vi "Interpret Opcode.vi"(10 "Opcode":u8 format="%x", 11 "Disassembler in":refnum<class "Disassembler.lvclass">) -> (1 "Addressing Mode":T2=enum."Immediate", 2 "Mnemonic":T1=enum."NOP", 3 "Disassembler out":refnum<class "Disassembler.lvclass">)   [LabVIEW 2021, in "Disassembler.lvclass"]
uses:
  Disassembler.lvclass
  Addressing Mode.ctl
  Menmonic.ctl
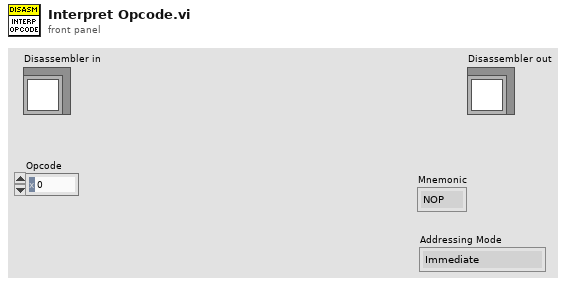
[diagram p1: front panel]
types:
  T1 = typedef "Disassembler.lvclass/Menmonic.ctl" = enum16{"Undefined", "ADC", "AND", "ASL", "BCC", "BCS", "BEQ", "BIT", "BMI", "BNE", "BPL", "BRK", "BVC", "BVS", "CLC", "CLD", "CLI", "CLV", "CMP", "CPX", "CPY", "DEC", "DEX", "DEY", "EOR", "INC", "INX", "INY", "JMP", "JSR", "LDA", "LDX", "LDY", "LSR", "NOP", "ORA", "PHA", "PHP", "PLA", "PLP", "ROL", "ROR", "RTI", "RTS", "SBC", "SEC", "SED", "SEI", "STA", "STX", "STY", "TAX", "TAY", "TSX", "TXA", "TXS", "TYA"}
  T2 = typedef "Disassembler.lvclass/Addressing Mode.ctl" = enum16{"Undefined", "Zero Page,Y", "Zero Page,X", "Zero Page", "Relative", "(indirect,X)", "(indirect),Y", "Implicit", "Immediate", "Accumulator", "Absolute,Y", "Absolute,X", "Absolute", "Indirect"}
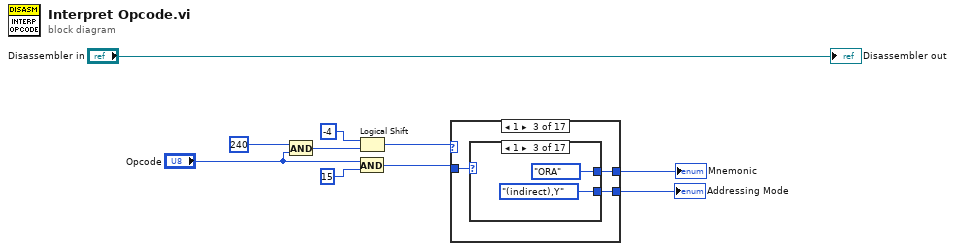
[diagram p0: block diagram]
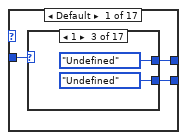
[diagram p2: hidden frame]
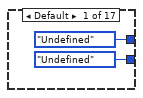
[diagram p3: hidden frame]
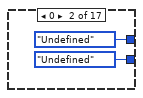
[diagram p4: hidden frame]
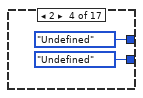
[diagram p5: hidden frame]
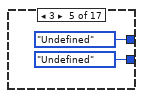
[diagram p6: hidden frame]
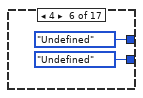
[diagram p7: hidden frame]
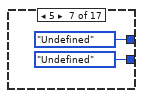
[diagram p8: hidden frame]
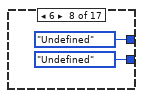
[diagram p9: hidden frame]
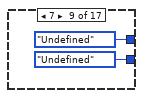
[diagram p10: hidden frame]
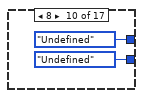
[diagram p11: hidden frame]
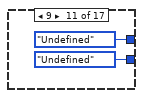
[diagram p12: hidden frame]
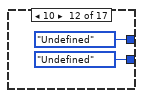
[diagram p13: hidden frame]
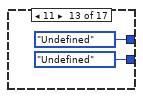
[diagram p14: hidden frame]
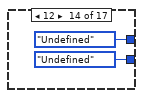
[diagram p15: hidden frame]
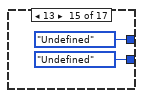
[diagram p16: hidden frame]
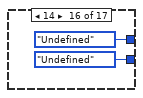
[diagram p17: hidden frame]
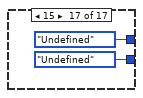
[diagram p18: hidden frame]
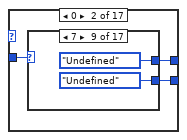
[diagram p19: hidden frame]
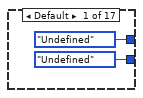
[diagram p20: hidden frame]
diagram:
  n1 = And(x=u8 240, y="Opcode") -> (x .and. y?=w8:u8)
  n2 = Logical Shift(y=i8 -4, x=w8) -> (x << y=w4:u8)
  n3 = And(x="Opcode", y=u8 15) -> (x .and. y?=w3:u8)
  n4 = case shown="1" w4 {
    tunnel: w3 -> [w13 w50 w87 w124 w161 w198 w235 w272 w309 w346 w383 w420 w457 w494 w531 w568 w605]
    tunnel: [w12 w49 w86 w123 w160 w197 w234 w271 w308 w345 w382 w419 w456 w493 w530 w567 w604] -> w2
    tunnel: [w11 w48 w85 w122 w159 w196 w233 w270 w307 w344 w381 w418 w455 w492 w529 w566 w603] -> w1
    frame Default {
      n5 = case shown="1" w13 {
        tunnel: [Menmonic."Undefined" Menmonic."Undefined" Menmonic."Undefined" Menmonic."Undefined" Menmonic."Undefined" Menmonic."Undefined" Menmonic."Undefined" Menmonic."Undefined" Menmonic."Undefined" Menmonic."Undefined" Menmonic."Undefined" Menmonic."Undefined" Menmonic."Undefined" Menmonic."Undefined" Menmonic."Undefined" Menmonic."Undefined" Menmonic."Undefined"] -> w12
        tunnel: [Addressing_Mode."Undefined" Addressing_Mode."Undefined" Addressing_Mode."Undefined" Addressing_Mode."Undefined" Addressing_Mode."Undefined" Addressing_Mode."Undefined" Addressing_Mode."Undefined" Addressing_Mode."Undefined" Addressing_Mode."Undefined" Addressing_Mode."Undefined" Addressing_Mode."Undefined" Addressing_Mode."Undefined" Addressing_Mode."Undefined" Addressing_Mode."Undefined" Addressing_Mode."Undefined" Addressing_Mode."Undefined" Addressing_Mode."Undefined"] -> w11
        frame Default {
        }
        frame 0 {
        }
        frame 1 {
        }
        frame 2 {
        }
        frame 3 {
        }
        frame 4 {
        }
        frame 5 {
        }
        frame 6 {
        }
        frame 7 {
        }
        frame 8 {
        }
        frame 9 {
        }
        frame 10 {
        }
        frame 11 {
        }
        frame 12 {
        }
        frame 13 {
        }
        frame 14 {
        }
        frame 15 {
        }
      }
    }
    frame 0 {
      n6 = case shown="7" w50 {
        tunnel: [Menmonic."Undefined" Menmonic."BRK" Menmonic."ORA" Menmonic."Undefined" Menmonic."Undefined" Menmonic."Undefined" Menmonic."ORA" Menmonic."ASL" Menmonic."Undefined" Menmonic."PHP" Menmonic."ORA" Menmonic."ASL" Menmonic."Undefined" Menmonic."Undefined" Menmonic."ORA" Menmonic."ASL" Menmonic."Undefined"] -> w49
        tunnel: [Addressing_Mode."Undefined" Addressing_Mode."Implicit" Addressing_Mode."(indirect,X)" Addressing_Mode."Undefined" Addressing_Mode."Undefined" Addressing_Mode."Undefined" Addressing_Mode."Zero Page" Addressing_Mode."Zero Page" Addressing_Mode."Undefined" Addressing_Mode."Implicit" Addressing_Mode."Immediate" Addressing_Mode."Accumulator" Addressing_Mode."Undefined" Addressing_Mode."Undefined" Addressing_Mode."Absolute" Addressing_Mode."Absolute" Addressing_Mode."Undefined"] -> w48
        frame Default {
        }
        frame 0 {
        }
        frame 1 {
        }
        frame 2 {
        }
        frame 3 {
        }
        frame 4 {
        }
        frame 5 {
        }
        frame 6 {
        }
        frame 7 {
        }
        frame 8 {
        }
        frame 9 {
        }
        frame 10 {
        }
        frame 11 {
        }
        frame 12 {
        }
        frame 13 {
        }
        frame 14 {
        }
        frame 15 {
        }
      }
    }
    frame 1 {
      n7 = case shown="1" w87 {
        tunnel: [Menmonic."Undefined" Menmonic."BPL" Menmonic."ORA" Menmonic."Undefined" Menmonic."Undefined" Menmonic."Undefined" Menmonic."ORA" Menmonic."ASL" Menmonic."Undefined" Menmonic."CLC" Menmonic."ORA" Menmonic."Undefined" Menmonic."Undefined" Menmonic."Undefined" Menmonic."ORA" Menmonic."ASL" Menmonic."Undefined"] -> w86
        tunnel: [Addressing_Mode."Undefined" Addressing_Mode."Relative" Addressing_Mode."(indirect),Y" Addressing_Mode."Undefined" Addressing_Mode."Undefined" Addressing_Mode."Undefined" Addressing_Mode."Zero Page,X" Addressing_Mode."Zero Page,X" Addressing_Mode."Undefined" Addressing_Mode."Implicit" Addressing_Mode."Absolute,Y" Addressing_Mode."Undefined" Addressing_Mode."Undefined" Addressing_Mode."Undefined" Addressing_Mode."Absolute,X" Addressing_Mode."Absolute,X" Addressing_Mode."Undefined"] -> w85
        frame Default {
        }
        frame 0 {
        }
        frame 1 {
        }
        frame 2 {
        }
        frame 3 {
        }
        frame 4 {
        }
        frame 5 {
        }
        frame 6 {
        }
        frame 7 {
        }
        frame 8 {
        }
        frame 9 {
        }
        frame 10 {
        }
        frame 11 {
        }
        frame 12 {
        }
        frame 13 {
        }
        frame 14 {
        }
        frame 15 {
        }
      }
    }
    frame 2 {
      n8 = case shown="E" w124 {
        tunnel: [Menmonic."Undefined" Menmonic."JSR" Menmonic."AND" Menmonic."Undefined" Menmonic."Undefined" Menmonic."BIT" Menmonic."AND" Menmonic."ROL" Menmonic."Undefined" Menmonic."PLP" Menmonic."AND" Menmonic."ROL" Menmonic."Undefined" Menmonic."BIT" Menmonic."AND" Menmonic."ROL" Menmonic."Undefined"] -> w123
        tunnel: [Addressing_Mode."Undefined" Addressing_Mode."Absolute" Addressing_Mode."(indirect,X)" Addressing_Mode."Undefined" Addressing_Mode."Undefined" Addressing_Mode."Zero Page" Addressing_Mode."Zero Page" Addressing_Mode."Zero Page" Addressing_Mode."Undefined" Addressing_Mode."Implicit" Addressing_Mode."Immediate" Addressing_Mode."Accumulator" Addressing_Mode."Undefined" Addressing_Mode."Absolute" Addressing_Mode."Absolute" Addressing_Mode."Absolute" Addressing_Mode."Undefined"] -> w122
        frame Default {
        }
        frame 0 {
        }
        frame 1 {
        }
        frame 2 {
        }
        frame 3 {
        }
        frame 4 {
        }
        frame 5 {
        }
        frame 6 {
        }
        frame 7 {
        }
        frame 8 {
        }
        frame 9 {
        }
        frame 10 {
        }
        frame 11 {
        }
        frame 12 {
        }
        frame 13 {
        }
        frame 14 {
        }
        frame 15 {
        }
      }
    }
    frame 3 {
      n9 = case shown="8" w161 {
        tunnel: [Menmonic."Undefined" Menmonic."BMI" Menmonic."AND" Menmonic."Undefined" Menmonic."Undefined" Menmonic."Undefined" Menmonic."AND" Menmonic."ROL" Menmonic."Undefined" Menmonic."SEC" Menmonic."AND" Menmonic."Undefined" Menmonic."Undefined" Menmonic."Undefined" Menmonic."AND" Menmonic."ROL" Menmonic."Undefined"] -> w160
        tunnel: [Addressing_Mode."Undefined" Addressing_Mode."Relative" Addressing_Mode."(indirect),Y" Addressing_Mode."Undefined" Addressing_Mode."Undefined" Addressing_Mode."Undefined" Addressing_Mode."Zero Page,X" Addressing_Mode."Zero Page,X" Addressing_Mode."Undefined" Addressing_Mode."Implicit" Addressing_Mode."Absolute,Y" Addressing_Mode."Undefined" Addressing_Mode."Undefined" Addressing_Mode."Undefined" Addressing_Mode."Absolute,X" Addressing_Mode."Absolute,X" Addressing_Mode."Undefined"] -> w159
        frame Default {
        }
        frame 0 {
        }
        frame 1 {
        }
        frame 2 {
        }
        frame 3 {
        }
        frame 4 {
        }
        frame 5 {
        }
        frame 6 {
        }
        frame 7 {
        }
        frame 8 {
        }
        frame 9 {
        }
        frame 10 {
        }
        frame 11 {
        }
        frame 12 {
        }
        frame 13 {
        }
        frame 14 {
        }
        frame 15 {
        }
      }
    }
    frame 4 {
      n10 = case shown="0" w198 {
        tunnel: [Menmonic."Undefined" Menmonic."RTI" Menmonic."EOR" Menmonic."Undefined" Menmonic."Undefined" Menmonic."Undefined" Menmonic."EOR" Menmonic."LSR" Menmonic."Undefined" Menmonic."PHA" Menmonic."EOR" Menmonic."LSR" Menmonic."Undefined" Menmonic."JMP" Menmonic."EOR" Menmonic."LSR" Menmonic."Undefined"] -> w197
        tunnel: [Addressing_Mode."Undefined" Addressing_Mode."Implicit" Addressing_Mode."(indirect,X)" Addressing_Mode."Undefined" Addressing_Mode."Undefined" Addressing_Mode."Undefined" Addressing_Mode."Zero Page" Addressing_Mode."Zero Page" Addressing_Mode."Undefined" Addressing_Mode."Implicit" Addressing_Mode."Immediate" Addressing_Mode."Accumulator" Addressing_Mode."Undefined" Addressing_Mode."Absolute" Addressing_Mode."Absolute" Addressing_Mode."Absolute" Addressing_Mode."Undefined"] -> w196
        frame Default {
        }
        frame 0 {
        }
        frame 1 {
        }
        frame 2 {
        }
        frame 3 {
        }
        frame 4 {
        }
        frame 5 {
        }
        frame 6 {
        }
        frame 7 {
        }
        frame 8 {
        }
        frame 9 {
        }
        frame 10 {
        }
        frame 11 {
        }
        frame 12 {
        }
        frame 13 {
        }
        frame 14 {
        }
        frame 15 {
        }
      }
    }
    frame 5 {
      n11 = case shown="E" w235 {
        tunnel: [Menmonic."Undefined" Menmonic."BVC" Menmonic."EOR" Menmonic."Undefined" Menmonic."Undefined" Menmonic."Undefined" Menmonic."EOR" Menmonic."LSR" Menmonic."Undefined" Menmonic."CLI" Menmonic."EOR" Menmonic."Undefined" Menmonic."Undefined" Menmonic."Undefined" Menmonic."EOR" Menmonic."LSR" Menmonic."Undefined"] -> w234
        tunnel: [Addressing_Mode."Undefined" Addressing_Mode."Relative" Addressing_Mode."(indirect),Y" Addressing_Mode."Undefined" Addressing_Mode."Undefined" Addressing_Mode."Undefined" Addressing_Mode."Zero Page,X" Addressing_Mode."Zero Page,X" Addressing_Mode."Undefined" Addressing_Mode."Implicit" Addressing_Mode."Absolute,Y" Addressing_Mode."Undefined" Addressing_Mode."Undefined" Addressing_Mode."Undefined" Addressing_Mode."Absolute,X" Addressing_Mode."Absolute,X" Addressing_Mode."Undefined"] -> w233
        frame Default {
        }
        frame 0 {
        }
        frame 1 {
        }
        frame 2 {
        }
        frame 3 {
        }
        frame 4 {
        }
        frame 5 {
        }
        frame 6 {
        }
        frame 7 {
        }
        frame 8 {
        }
        frame 9 {
        }
        frame 10 {
        }
        frame 11 {
        }
        frame 12 {
        }
        frame 13 {
        }
        frame 14 {
        }
        frame 15 {
        }
      }
    }
    frame 6 {
      n12 = case shown="C" w272 {
        tunnel: [Menmonic."Undefined" Menmonic."RTS" Menmonic."ADC" Menmonic."Undefined" Menmonic."Undefined" Menmonic."Undefined" Menmonic."ADC" Menmonic."ROR" Menmonic."Undefined" Menmonic."PLA" Menmonic."ADC" Menmonic."ROR" Menmonic."Undefined" Menmonic."JMP" Menmonic."ADC" Menmonic."ROR" Menmonic."Undefined"] -> w271
        tunnel: [Addressing_Mode."Undefined" Addressing_Mode."Implicit" Addressing_Mode."(indirect,X)" Addressing_Mode."Undefined" Addressing_Mode."Undefined" Addressing_Mode."Undefined" Addressing_Mode."Zero Page" Addressing_Mode."Zero Page" Addressing_Mode."Undefined" Addressing_Mode."Implicit" Addressing_Mode."Immediate" Addressing_Mode."Accumulator" Addressing_Mode."Undefined" Addressing_Mode."Indirect" Addressing_Mode."Absolute" Addressing_Mode."Absolute" Addressing_Mode."Undefined"] -> w270
        frame Default {
        }
        frame 0 {
        }
        frame 1 {
        }
        frame 2 {
        }
        frame 3 {
        }
        frame 4 {
        }
        frame 5 {
        }
        frame 6 {
        }
        frame 7 {
        }
        frame 8 {
        }
        frame 9 {
        }
        frame 10 {
        }
        frame 11 {
        }
        frame 12 {
        }
        frame 13 {
        }
        frame 14 {
        }
        frame 15 {
        }
      }
    }
    frame 7 {
      n13 = case shown="C" w309 {
        tunnel: [Menmonic."Undefined" Menmonic."BVS" Menmonic."ADC" Menmonic."Undefined" Menmonic."Undefined" Menmonic."Undefined" Menmonic."ADC" Menmonic."ROR" Menmonic."Undefined" Menmonic."SEI" Menmonic."ADC" Menmonic."Undefined" Menmonic."Undefined" Menmonic."Undefined" Menmonic."ADC" Menmonic."ROR" Menmonic."Undefined"] -> w308
        tunnel: [Addressing_Mode."Undefined" Addressing_Mode."Relative" Addressing_Mode."(indirect),Y" Addressing_Mode."Undefined" Addressing_Mode."Undefined" Addressing_Mode."Undefined" Addressing_Mode."Zero Page,X" Addressing_Mode."Zero Page,X" Addressing_Mode."Undefined" Addressing_Mode."Implicit" Addressing_Mode."Absolute,Y" Addressing_Mode."Undefined" Addressing_Mode."Undefined" Addressing_Mode."Undefined" Addressing_Mode."Absolute,X" Addressing_Mode."Absolute,X" Addressing_Mode."Undefined"] -> w307
        frame Default {
        }
        frame 0 {
        }
        frame 1 {
        }
        frame 2 {
        }
        frame 3 {
        }
        frame 4 {
        }
        frame 5 {
        }
        frame 6 {
        }
        frame 7 {
        }
        frame 8 {
        }
        frame 9 {
        }
        frame 10 {
        }
        frame 11 {
        }
        frame 12 {
        }
        frame 13 {
        }
        frame 14 {
        }
        frame 15 {
        }
      }
    }
    frame 8 {
      n14 = case shown="D" w346 {
        tunnel: [Menmonic."Undefined" Menmonic."Undefined" Menmonic."STA" Menmonic."Undefined" Menmonic."Undefined" Menmonic."STY" Menmonic."STA" Menmonic."STX" Menmonic."Undefined" Menmonic."DEY" Menmonic."Undefined" Menmonic."TXA" Menmonic."Undefined" Menmonic."STY" Menmonic."STA" Menmonic."STX" Menmonic."Undefined"] -> w345
        tunnel: [Addressing_Mode."Undefined" Addressing_Mode."Undefined" Addressing_Mode."(indirect,X)" Addressing_Mode."Undefined" Addressing_Mode."Undefined" Addressing_Mode."Zero Page" Addressing_Mode."Zero Page" Addressing_Mode."Zero Page" Addressing_Mode."Undefined" Addressing_Mode."Implicit" Addressing_Mode."Undefined" Addressing_Mode."Implicit" Addressing_Mode."Undefined" Addressing_Mode."Absolute" Addressing_Mode."Absolute" Addressing_Mode."Absolute" Addressing_Mode."Undefined"] -> w344
        frame Default {
        }
        frame 0 {
        }
        frame 1 {
        }
        frame 2 {
        }
        frame 3 {
        }
        frame 4 {
        }
        frame 5 {
        }
        frame 6 {
        }
        frame 7 {
        }
        frame 8 {
        }
        frame 9 {
        }
        frame 10 {
        }
        frame 11 {
        }
        frame 12 {
        }
        frame 13 {
        }
        frame 14 {
        }
        frame 15 {
        }
      }
    }
    frame 9 {
      n15 = case shown="8" w383 {
        tunnel: [Menmonic."Undefined" Menmonic."BCC" Menmonic."STA" Menmonic."Undefined" Menmonic."Undefined" Menmonic."STY" Menmonic."STA" Menmonic."STX" Menmonic."Undefined" Menmonic."TYA" Menmonic."STA" Menmonic."TXS" Menmonic."Undefined" Menmonic."Undefined" Menmonic."STA" Menmonic."Undefined" Menmonic."Undefined"] -> w382
        tunnel: [Addressing_Mode."Undefined" Addressing_Mode."Relative" Addressing_Mode."(indirect),Y" Addressing_Mode."Undefined" Addressing_Mode."Undefined" Addressing_Mode."Zero Page,X" Addressing_Mode."Zero Page,X" Addressing_Mode."Zero Page,Y" Addressing_Mode."Undefined" Addressing_Mode."Implicit" Addressing_Mode."Absolute,Y" Addressing_Mode."Implicit" Addressing_Mode."Undefined" Addressing_Mode."Undefined" Addressing_Mode."Absolute,X" Addressing_Mode."Undefined" Addressing_Mode."Undefined"] -> w381
        frame Default {
        }
        frame 0 {
        }
        frame 1 {
        }
        frame 2 {
        }
        frame 3 {
        }
        frame 4 {
        }
        frame 5 {
        }
        frame 6 {
        }
        frame 7 {
        }
        frame 8 {
        }
        frame 9 {
        }
        frame 10 {
        }
        frame 11 {
        }
        frame 12 {
        }
        frame 13 {
        }
        frame 14 {
        }
        frame 15 {
        }
      }
    }
    frame 10 {
      n16 = case shown="1" w420 {
        tunnel: [Menmonic."Undefined" Menmonic."LDY" Menmonic."LDA" Menmonic."LDX" Menmonic."Undefined" Menmonic."LDY" Menmonic."LDA" Menmonic."LDX" Menmonic."Undefined" Menmonic."TAY" Menmonic."LDA" Menmonic."TAX" Menmonic."Undefined" Menmonic."LDY" Menmonic."LDA" Menmonic."LDX" Menmonic."Undefined"] -> w419
        tunnel: [Addressing_Mode."Undefined" Addressing_Mode."Immediate" Addressing_Mode."(indirect,X)" Addressing_Mode."Immediate" Addressing_Mode."Undefined" Addressing_Mode."Zero Page" Addressing_Mode."Zero Page" Addressing_Mode."Zero Page" Addressing_Mode."Undefined" Addressing_Mode."Implicit" Addressing_Mode."Immediate" Addressing_Mode."Implicit" Addressing_Mode."Undefined" Addressing_Mode."Absolute" Addressing_Mode."Absolute" Addressing_Mode."Absolute" Addressing_Mode."Undefined"] -> w418
        frame Default {
        }
        frame 0 {
        }
        frame 1 {
        }
        frame 2 {
        }
        frame 3 {
        }
        frame 4 {
        }
        frame 5 {
        }
        frame 6 {
        }
        frame 7 {
        }
        frame 8 {
        }
        frame 9 {
        }
        frame 10 {
        }
        frame 11 {
        }
        frame 12 {
        }
        frame 13 {
        }
        frame 14 {
        }
        frame 15 {
        }
      }
    }
    frame 11 {
      n17 = case shown="A" w457 {
        tunnel: [Menmonic."Undefined" Menmonic."BCS" Menmonic."LDA" Menmonic."Undefined" Menmonic."Undefined" Menmonic."LDY" Menmonic."LDA" Menmonic."LDX" Menmonic."Undefined" Menmonic."CLV" Menmonic."LDA" Menmonic."TSX" Menmonic."Undefined" Menmonic."LDY" Menmonic."LDA" Menmonic."LDX" Menmonic."Undefined"] -> w456
        tunnel: [Addressing_Mode."Undefined" Addressing_Mode."Relative" Addressing_Mode."(indirect),Y" Addressing_Mode."Undefined" Addressing_Mode."Undefined" Addressing_Mode."Zero Page,X" Addressing_Mode."Zero Page,X" Addressing_Mode."Zero Page,Y" Addressing_Mode."Undefined" Addressing_Mode."Implicit" Addressing_Mode."Absolute,Y" Addressing_Mode."Implicit" Addressing_Mode."Undefined" Addressing_Mode."Absolute,X" Addressing_Mode."Absolute,X" Addressing_Mode."Absolute,Y" Addressing_Mode."Undefined"] -> w455
        frame Default {
        }
        frame 0 {
        }
        frame 1 {
        }
        frame 2 {
        }
        frame 3 {
        }
        frame 4 {
        }
        frame 5 {
        }
        frame 6 {
        }
        frame 7 {
        }
        frame 8 {
        }
        frame 9 {
        }
        frame 10 {
        }
        frame 11 {
        }
        frame 12 {
        }
        frame 13 {
        }
        frame 14 {
        }
        frame 15 {
        }
      }
    }
    frame 12 {
      n18 = case shown="4" w494 {
        tunnel: [Menmonic."Undefined" Menmonic."CPY" Menmonic."CMP" Menmonic."Undefined" Menmonic."Undefined" Menmonic."CPY" Menmonic."CMP" Menmonic."DEC" Menmonic."Undefined" Menmonic."INY" Menmonic."CMP" Menmonic."DEX" Menmonic."Undefined" Menmonic."CPY" Menmonic."CMP" Menmonic."DEC" Menmonic."Undefined"] -> w493
        tunnel: [Addressing_Mode."Undefined" Addressing_Mode."Immediate" Addressing_Mode."(indirect,X)" Addressing_Mode."Undefined" Addressing_Mode."Undefined" Addressing_Mode."Zero Page" Addressing_Mode."Zero Page" Addressing_Mode."Zero Page" Addressing_Mode."Undefined" Addressing_Mode."Implicit" Addressing_Mode."Immediate" Addressing_Mode."Implicit" Addressing_Mode."Undefined" Addressing_Mode."Absolute" Addressing_Mode."Absolute" Addressing_Mode."Absolute" Addressing_Mode."Undefined"] -> w492
        frame Default {
        }
        frame 0 {
        }
        frame 1 {
        }
        frame 2 {
        }
        frame 3 {
        }
        frame 4 {
        }
        frame 5 {
        }
        frame 6 {
        }
        frame 7 {
        }
        frame 8 {
        }
        frame 9 {
        }
        frame 10 {
        }
        frame 11 {
        }
        frame 12 {
        }
        frame 13 {
        }
        frame 14 {
        }
        frame 15 {
        }
      }
    }
    frame 13 {
      n19 = case shown="8" w531 {
        tunnel: [Menmonic."Undefined" Menmonic."BNE" Menmonic."CMP" Menmonic."Undefined" Menmonic."Undefined" Menmonic."Undefined" Menmonic."CMP" Menmonic."DEC" Menmonic."Undefined" Menmonic."CLD" Menmonic."CMP" Menmonic."Undefined" Menmonic."Undefined" Menmonic."Undefined" Menmonic."CMP" Menmonic."DEC" Menmonic."Undefined"] -> w530
        tunnel: [Addressing_Mode."Undefined" Addressing_Mode."Relative" Addressing_Mode."(indirect),Y" Addressing_Mode."Undefined" Addressing_Mode."Undefined" Addressing_Mode."Undefined" Addressing_Mode."Zero Page,X" Addressing_Mode."Zero Page,X" Addressing_Mode."Undefined" Addressing_Mode."Implicit" Addressing_Mode."Absolute,Y" Addressing_Mode."Undefined" Addressing_Mode."Undefined" Addressing_Mode."Undefined" Addressing_Mode."Absolute,X" Addressing_Mode."Absolute,X" Addressing_Mode."Undefined"] -> w529
        frame Default {
        }
        frame 0 {
        }
        frame 1 {
        }
        frame 2 {
        }
        frame 3 {
        }
        frame 4 {
        }
        frame 5 {
        }
        frame 6 {
        }
        frame 7 {
        }
        frame 8 {
        }
        frame 9 {
        }
        frame 10 {
        }
        frame 11 {
        }
        frame 12 {
        }
        frame 13 {
        }
        frame 14 {
        }
        frame 15 {
        }
      }
    }
    frame 14 {
      n20 = case shown="E" w568 {
        tunnel: [Menmonic."Undefined" Menmonic."CPX" Menmonic."SBC" Menmonic."Undefined" Menmonic."Undefined" Menmonic."CPX" Menmonic."SBC" Menmonic."INC" Menmonic."Undefined" Menmonic."INX" Menmonic."SBC" Menmonic."NOP" Menmonic."Undefined" Menmonic."CPX" Menmonic."SBC" Menmonic."INC" Menmonic."Undefined"] -> w567
        tunnel: [Addressing_Mode."Undefined" Addressing_Mode."Immediate" Addressing_Mode."(indirect,X)" Addressing_Mode."Undefined" Addressing_Mode."Undefined" Addressing_Mode."Zero Page" Addressing_Mode."Zero Page" Addressing_Mode."Zero Page" Addressing_Mode."Undefined" Addressing_Mode."Implicit" Addressing_Mode."Immediate" Addressing_Mode."Implicit" Addressing_Mode."Undefined" Addressing_Mode."Absolute" Addressing_Mode."Absolute" Addressing_Mode."Absolute" Addressing_Mode."Undefined"] -> w566
        frame Default {
        }
        frame 0 {
        }
        frame 1 {
        }
        frame 2 {
        }
        frame 3 {
        }
        frame 4 {
        }
        frame 5 {
        }
        frame 6 {
        }
        frame 7 {
        }
        frame 8 {
        }
        frame 9 {
        }
        frame 10 {
        }
        frame 11 {
        }
        frame 12 {
        }
        frame 13 {
        }
        frame 14 {
        }
        frame 15 {
        }
      }
    }
    frame 15 {
      n21 = case shown="8" w605 {
        tunnel: [Menmonic."Undefined" Menmonic."BEQ" Menmonic."SBC" Menmonic."Undefined" Menmonic."Undefined" Menmonic."Undefined" Menmonic."SBC" Menmonic."INC" Menmonic."Undefined" Menmonic."SED" Menmonic."SBC" Menmonic."Undefined" Menmonic."Undefined" Menmonic."Undefined" Menmonic."SBC" Menmonic."INC" Menmonic."Undefined"] -> w604
        tunnel: [Addressing_Mode."Undefined" Addressing_Mode."Relative" Addressing_Mode."(indirect),Y" Addressing_Mode."Undefined" Addressing_Mode."Undefined" Addressing_Mode."Undefined" Addressing_Mode."Zero Page,X" Addressing_Mode."Zero Page,X" Addressing_Mode."Undefined" Addressing_Mode."Implicit" Addressing_Mode."Absolute,Y" Addressing_Mode."Undefined" Addressing_Mode."Undefined" Addressing_Mode."Undefined" Addressing_Mode."Absolute,X" Addressing_Mode."Absolute,X" Addressing_Mode."Undefined"] -> w603
        frame Default {
        }
        frame 0 {
        }
        frame 1 {
        }
        frame 2 {
        }
        frame 3 {
        }
        frame 4 {
        }
        frame 5 {
        }
        frame 6 {
        }
        frame 7 {
        }
        frame 8 {
        }
        frame 9 {
        }
        frame 10 {
        }
        frame 11 {
        }
        frame 12 {
        }
        frame 13 {
        }
        frame 14 {
        }
        frame 15 {
        }
      }
    }
  }
  "Addressing Mode" <- w1
  "Mnemonic" <- w2
  "Disassembler out" <- "Disassembler in"
